vi "Decide next action.vi"(7 "Polarization-based seek? (F)":bool, 8 "error in (no error)":errorcluster, 9 "\"Good\" rate threshold":dbl, 10 "Seek positive polarization?":bool, 11 "Automatic Mode in":refnum<class "Automatic Mode.lvclass">) -> (0 "error out":errorcluster, 1 "Calculated rate":dbl, 2 "Decision":T1, 3 "Automatic Mode out":refnum<class "Automatic Mode.lvclass">)   [LabVIEW 2015, in "Automatic Mode.lvclass"]
uses:
  Automatic Mode.lvclass
  Controller decision.ctl
  Automatic Mode.lvclass/Automatic Mode.ctl
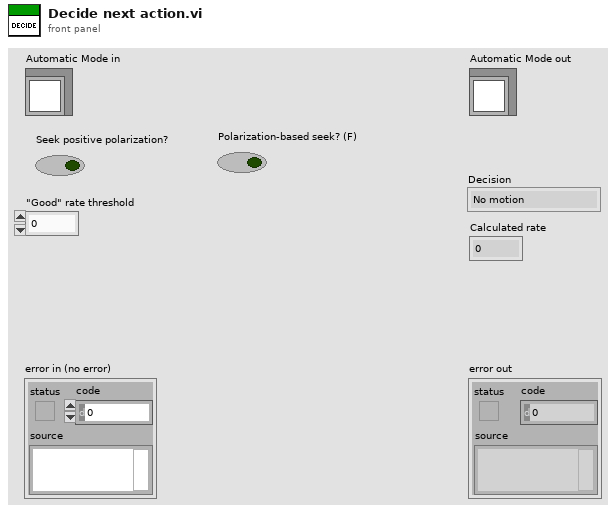
[diagram p1: front panel]
types:
  T1 = typedef "Controller decision.ctl" = enum16{"No motion", "Switch direction", "Keep current direction"}
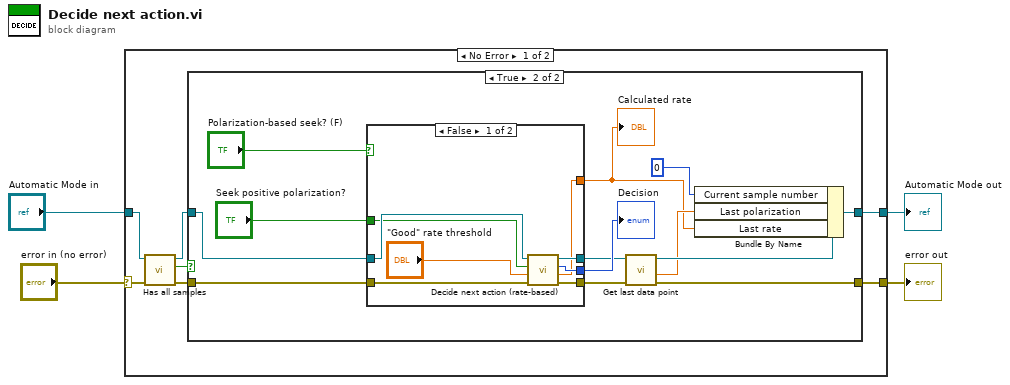
[diagram p0: block diagram]
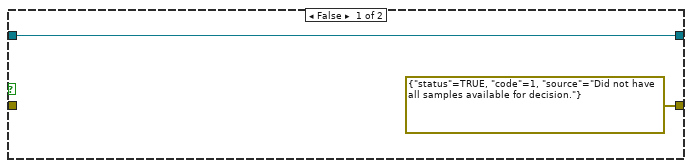
[diagram p2: hidden frame]
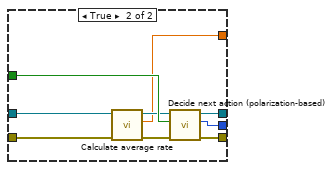
[diagram p3: hidden frame]
diagram:
  n1 = case shown="No Error" "error in (no error)" {
    selector: "error in (no error)" -> [w9 w45]
    tunnel: [w7 w45] -> w3
    tunnel: [w5 w44] -> w1
    tunnel: "Automatic Mode in" -> [w11 w44]
    frame No Error {
      n2 = call "Has all samples.vi"("error in (no error)"=w9, "Automatic Mode in"=w11) -> ("error out"=w8:errorcluster, "Has all samples?"=w10:bool, "Automatic Mode out"=w6:refnum<class "Automatic Mode.lvclass">)  [unwired: 7 in]
      n3 = case shown="True" w10 {
        tunnel: w8 -> [_ w15]
        tunnel: [errorcluster {"status"=TRUE, "code"=1, "source"="Did not have all samples available for decision."} ("error out") w18] -> w7
        tunnel: w6 -> [w12 w16]
        tunnel: [w12 w26] -> w5
        frame False {
        }
        frame True {
          n4 = case shown="False" "Polarization-based seek? (F)" {
            tunnel: w16 -> [w33 w36]
            tunnel: w15 -> [w34 w39]
            tunnel: "Seek positive polarization?" -> [w27 w43]
            tunnel: [w32 w42] -> w21
            tunnel: [w31 w41] -> w22
            tunnel: [w29 w40] -> w19
            tunnel: [w30 w35] -> w14
            frame False {
              n5 = call "Decide next action (rate-based).vi"("error in (no error)"=w34, "\"Good\" rate threshold"="\"Good\" rate threshold", "Seek positive polarization?"=w27, "Automatic Mode in"=w33) -> ("error out"=w29:errorcluster, "New rate"=w30:dbl, "Decision"=w31:T1, "Automatic Mode out"=w32:refnum<class "Automatic Mode.lvclass">)  [unwired: 4 in]
            }
            frame True {
              n6 = call "Calculate average rate.vi"("error in (no error)"=w39, "Automatic Mode in"=w36) -> ("error out"=w38:errorcluster, "Average rate"=w35:dbl, "Automatic Mode out"=w37:refnum<class "Automatic Mode.lvclass">)  [unwired: 7 in]
              n7 = call "Decide next action (polarization-based).vi"("error in (no error)"=w38, "Seek positive polarization?"=w43, "Automatic Mode in"=w37) -> ("error out"=w40:errorcluster, "Decision"=w41:T1, "Automatic Mode out"=w42:refnum<class "Automatic Mode.lvclass">)  [unwired: 6 in]
            }
          }
          "Decision" <- w22
          "Calculated rate" <- w14
          n8 = call "Get last data point.vi"("error in (no error)"=w19, "Automatic Mode in"=w21) -> ("error out"=w18:errorcluster, "Polarization"=w17:dbl, "Automatic Mode out"=w20:refnum<class "Automatic Mode.lvclass">)  [unwired: 6 in, 1 out]
          n9 = Bundle By Name(cluster=w20, "Current sample number"=0, "Last polarization"=w17, "Last rate"=w14) -> (w26:refnum<class "Automatic Mode.lvclass">)
        }
      }
    }
    frame Error {
    }
  }
  "error out" <- w3
  "Automatic Mode out" <- w1
